vi "Open Close Valves.vi"(0 "Valves to Open":i32[](array[numeric]), 1 "Valves to Close":i32[](array[numeric]), 3 "Emergency Stop":bool, 5 "Current Valve State":refnum<vi>, 6 "Debug Mode":refnum<vi>, 7 "Reactor Name":string=" and close valves: ", 8 "Reactor Selector":T1(ring), 10 "Pump Valves":i32[](array[numeric]), 11 "System Queue":refnum<vi>, 13 "JSON Queue":refnum<vi>) -> ()   [LabVIEW 2022 SP3]
uses:
  <vilib>/Utility/error.llb/whitespace.ctl
  <vilib>/Utility/error.llb/Trim Whitespace One-Sided.vi
panel:
  out "Array":bool[](array[boolean])
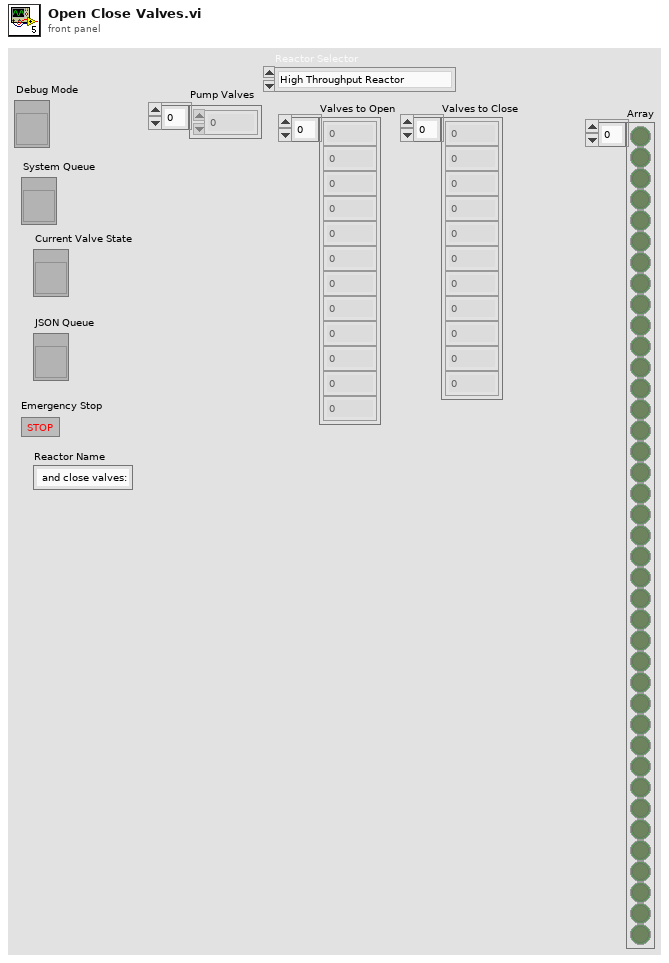
[diagram p1: front panel]
types:
  T1 = enum16{"High Throughput Reactor", "In Situ Reactor", "MLD Reactor"}
  T2 = cluster{"type":string, "meta":string, "payload":cluster{"LogMessage":string, "reactorName":string, "timeStamp":string}}
  T3 = cluster{"LogMessage":string, "timeStamp":string, "reactorName":string}
  T4 = typedef "whitespace.ctl" = u16
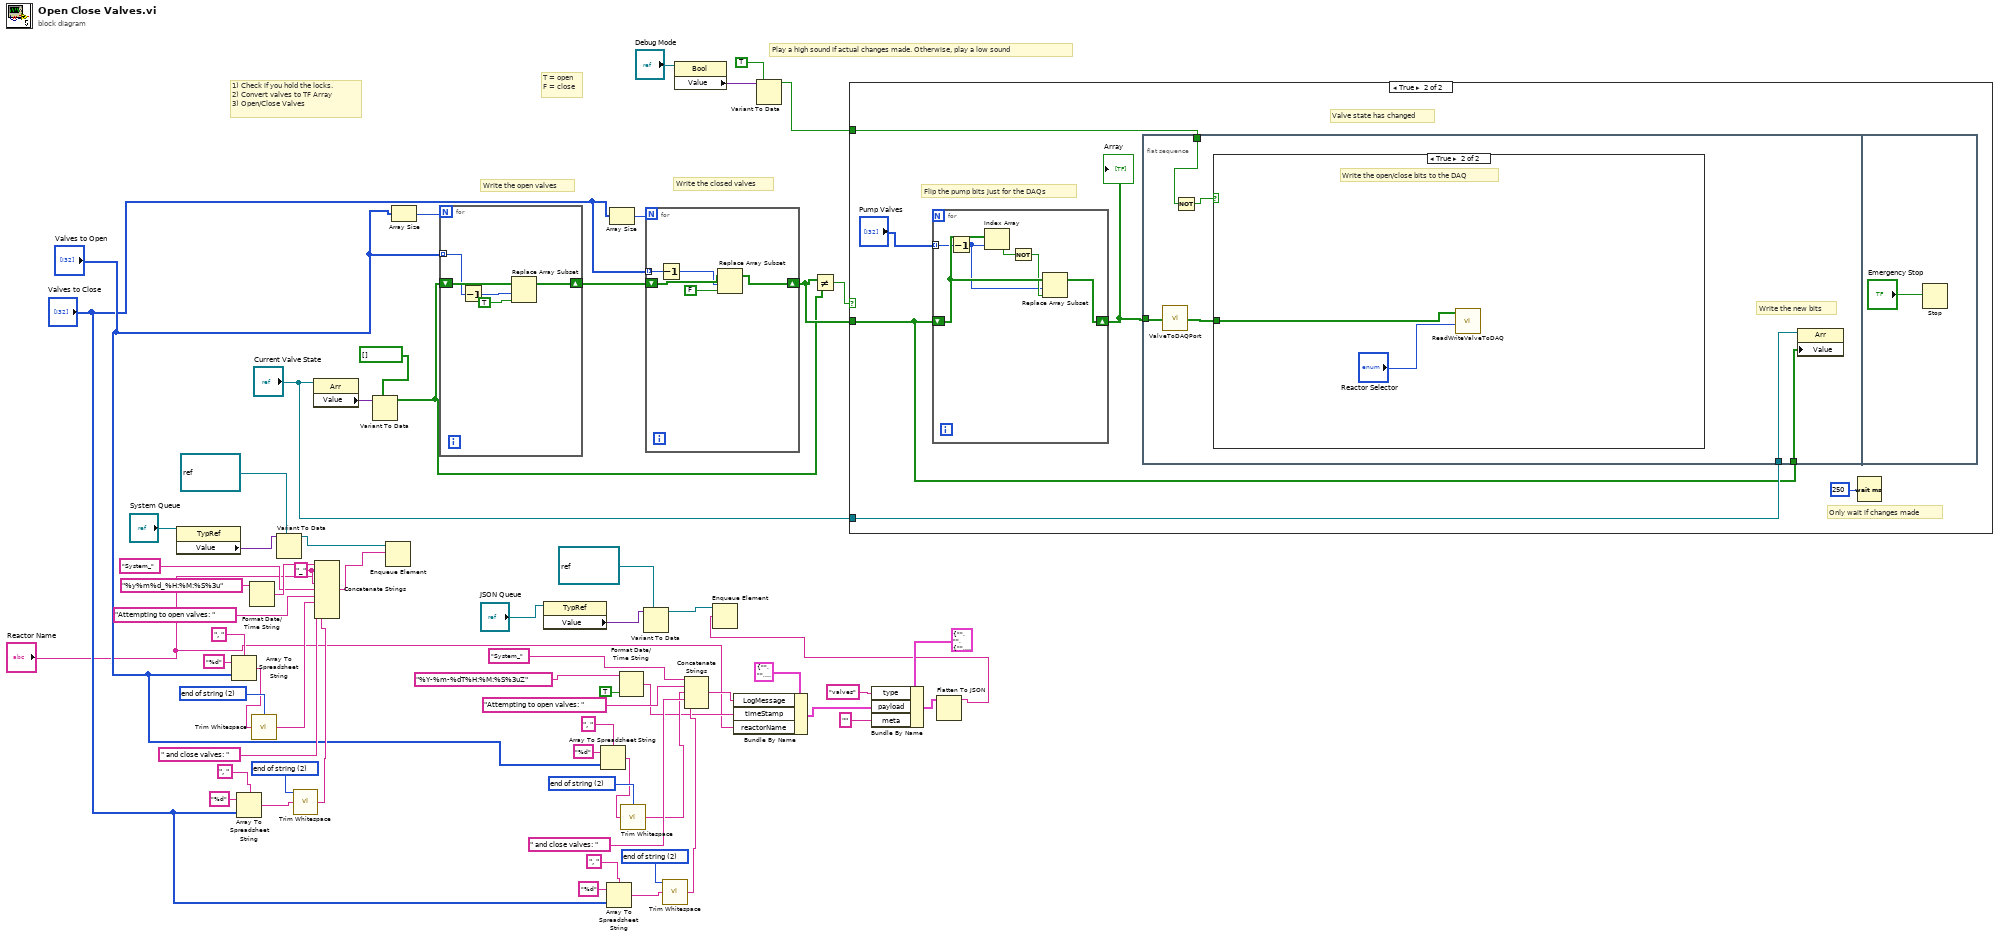
[diagram p0: block diagram]
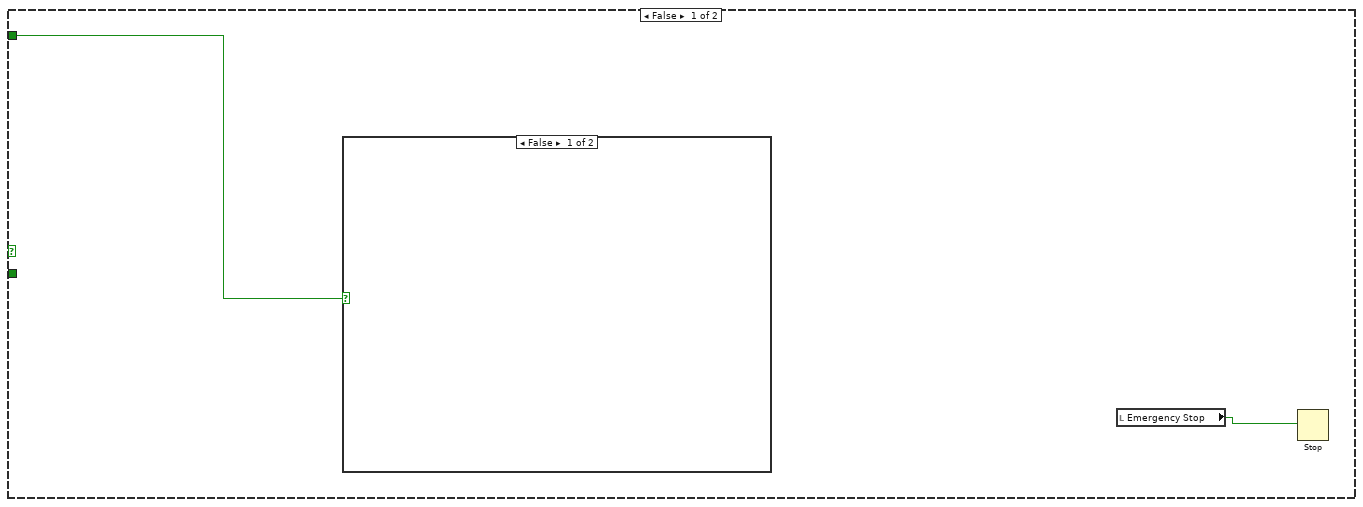
[diagram p2: hidden frame]
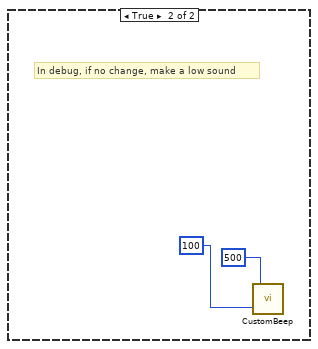
[diagram p3: hidden frame]
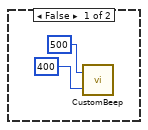
[diagram p4: hidden frame]
diagram:
  w5 = "_" ("string")
  w25 = T4 2 items=["both", "start of string", "end of string"] ("location (both)")
  w30 = T4 2 items=["both", "start of string", "end of string"] ("location (both)")
  w43 = T4 2 items=["both", "start of string", "end of string"] ("location (both)")
  w48 = T4 2 items=["both", "start of string", "end of string"] ("location (both)")
  # "Play a high sound if actual changes made. Otherwise, play a low sound"
  # "Write the closed valves"
  # "Write the open valves"
  # "T = open\nF = close"
  # "1) Check if you hold the locks.\n2) Convert valves to TF Array\n3) Open/Close Valves"
  n1 = property class="TypRef"(reference="System Queue") -> ("Value"=w50:variant)  [unwired: 1 in, 2 out]
  n2 = Array To Spreadsheet String(delimiter (Tab)=", ", array="Valves to Open", 3:"%d" ("format string")) -> (spreadsheet string=w47:string)
  n3 = Array To Spreadsheet String(delimiter (Tab)=", ", array="Valves to Close", 3:"%d" ("format string")) -> (spreadsheet string=w44:string)
  n4 = Format Date/Time String(time format string (%c)="%y%m%d_%H:%M:%S%3u") -> (date/time string=w6:string)  [unwired: 2 in]
  n5 = call <vilib>:"Trim Whitespace.vi"("string"=w47, "location (both)"=w48) -> ("trimmed string"=w46:string)
  n6 = Variant To Data(type=refnum<queue> refnum ("Queue Reactor 6"), Variant=w50) -> (data=w49:refnum<queue>)  [unwired: 1 in, 1 out]
  n7 = call <vilib>:"Trim Whitespace.vi"("string"=w44, "location (both)"=w43) -> ("trimmed string"=w45:string)
  n8 = property class="Arr"(reference="Current Valve State") -> ("Value"=w40:variant)  [unwired: 1 in, 2 out]
  n9 = Concatenate Strings(w6, w5, "Reactor Name", w5, "System_" ("string"), "Attempting to open valves: " ("element"), w46, " and close valves: " ("element"), w45) -> (w53:string)
  n10 = Variant To Data(type=bool[] [], Variant=w40) -> (data=w8:bool[])  [unwired: 1 in, 1 out]
  n11 = Enqueue Element(queue=w49, element=w53) -> ()  [unwired: 2 in, 3 out]
  n12 = Array Size(array="Valves to Open") -> (size(s)=w65:i32)
  n13 = for {
    N: w65 -> [_]
    tunnel: "Valves to Open" -> [w68] mode=indexing
    shift-right: [w70] -> w62
    shift-left: w8 -> [w69]
    n14 = Decrement(x=w68) -> (x-1=w66:i32)
    n15 = Replace Array Subset(array=w69, new element=TRUE ("new element/subarray"), index=w66) -> (w70:bool[])
  }
  n16 = property class="TypRef"(reference="JSON Queue") -> ("Value"=w39:variant)  [unwired: 1 in, 2 out]
  n17 = Array To Spreadsheet String(delimiter (Tab)=", ", array="Valves to Open", 3:"%d" ("format string")) -> (spreadsheet string=w29:string)
  n18 = Array To Spreadsheet String(delimiter (Tab)=", ", array="Valves to Close", 3:"%d" ("format string")) -> (spreadsheet string=w26:string)
  n19 = Array Size(array="Valves to Close") -> (size(s)=w63:i32)
  n20 = Format Date/Time String(time format string (%c)="%Y-%m-%dT%H:%M:%S%3uZ", UTC format=TRUE) -> (date/time string=w3:string)  [unwired: 1 in]
  n21 = call <vilib>:"Trim Whitespace.vi"("string"=w29, "location (both)"=w30) -> ("trimmed string"=w28:string)
  n22 = Variant To Data(type=refnum<queue> refnum ("Queue Reactor 6"), Variant=w39) -> (data=w38:refnum<queue>)  [unwired: 1 in, 1 out]
  n23 = for {
    N: w63 -> [_]
    tunnel: "Valves to Close" -> [w74] mode=indexing
    shift-right: [w72] -> w9
    shift-left: w62 -> [w73]
    n24 = Decrement(x=w74) -> (x-1=w71:i32)
    n25 = Replace Array Subset(array=w73, new element=FALSE ("new element/subarray"), index=w71) -> (w72:bool[])
  }
  n26 = call <vilib>:"Trim Whitespace.vi"("string"=w26, "location (both)"=w25) -> ("trimmed string"=w27:string)
  n27 = property class="Bool"(reference="Debug Mode") -> ("Value"=w12:variant)  [unwired: 1 in, 2 out]
  n28 = Concatenate Strings("System_" ("string"), "Attempting to open valves: " ("element"), w28, " and close valves: " ("element"), w27) -> (w20:string)
  n29 = Bundle By Name(cluster=T3 {"LogMessage"="", "timeStamp"="", "reactorName"=""} ("input cluster"), "LogMessage"=w20, "timeStamp"=w3, "reactorName"="Reactor Name") -> (w18:T3)
  n30 = Variant To Data(type=TRUE, Variant=w12) -> (data=w10:bool)  [unwired: 1 in, 1 out]
  n31 = Not Equal?(x=w9, y=w8) -> (x != y?=w7:bool)
  n32 = case shown="True" w7 {
    tunnel: "Current Valve State" -> [_ w85]
    tunnel: w10 -> [w76 w82]
    tunnel: w9 -> [_ w81]
    frame False {
      n33 = case shown="False" w76 {
        frame False {
        }
        frame True {
          # "In debug, if no change, make a low sound"
          n34 = call "CustomBeep.vi"("Frequency"=u32 100 ("frequency (Hz)"), "Approx Duration (ms)"=u32 500 ("duration (msec)")) -> ()  [unwired: 1 in]
        }
      }
      n35 = local read "Emergency Stop"() -> (w77:bool)
      n36 = Stop(stop? (T)=w77) -> ()
    }
    frame True {
      # "Only wait if changes made"
      # "Valve state has changed"
      # "Flip the pump bits just for the DAQs"
      n37 = for {
        tunnel: "Pump Valves" -> [w101] mode=indexing
        shift-right: [w98] -> w83
        shift-left: w81 -> [w102]
        n38 = Decrement(x=w101) -> (x-1=w97:i32)
        n39 = Index Array(array=w102, index=w97) -> (element=w100:bool)
        n40 = Not(x=w100) -> (.not. x?=w99:bool)
        n41 = Replace Array Subset(array=w102, new element=w99, index=w97) -> (w98:bool[])
      }
      "Array" <- w83
      n42 = flat-sequence {
        tunnel: w85 -> [w91]
        tunnel: w81 -> [w90]
        tunnel: w83 -> [w86]
        tunnel: w82 -> [w87]
        frame #0 {
          # "Write the new bits"
          n43 = call "ValveToDAQPort.vi"("Valves"=w86) -> ("DAQ Ports"=w89:bool[])
          n44 = Not(x=w87) -> (.not. x?=w88:bool)
          n45 = case shown="True" w88 {
            tunnel: w89 -> [_ w95]
            frame False {
              n46 = call "CustomBeep.vi"("Frequency"=u32 400 ("frequency (Hz)"), "Approx Duration (ms)"=u32 500 ("duration (msec)")) -> ()  [unwired: 1 in]
            }
            frame True {
              # "Write the open/close bits to the DAQ"
              n47 = call "ReadWriteValveToDAQ.vi"("Reactor Selector"="Reactor Selector", "DAQ Ports"=w95) -> ()  [unwired: 10 in]
            }
          }
          n48 = property class="Arr"(reference=w91, "Value"=w90) -> ()  [unwired: 1 in, 2 out]
        }
        frame #1 {
          n49 = Stop(stop? (T)="Emergency Stop") -> ()
        }
      }
      n50 = Wait (ms)(milliseconds to wait=u32 250) -> ()  [unwired: 1 out]
    }
  }
  n51 = Bundle By Name(cluster=T2 {"type"="", "meta"="", "payload"={"LogMessage"="", "reactorName"="", "timeStamp"=""}} ("input cluster"), "type"="valves", "payload"=w18, "meta"="") -> (w15:T2)
  n52 = Flatten To JSON(anything=w15) -> (JSON string=w14:string)  [unwired: 2 in, 1 out]
  n53 = Enqueue Element(queue=w38, element=w14) -> ()  [unwired: 2 in, 3 out]
